vi "FTW-TestExecutive-Sequence-Serialize.vi"(0 "Sequence":T1[](array[typedef]) {"Results"."Start Time" format="%<%Y-%m-%d %H:%M:%S%03u>T"; "Results"."Elapsed Time" format="%<%H:%M:%S%3u>t"; "Elapsed Time" format="%<%H:%M:%S%3u>t"}, 11 "error in":errorcluster) -> (4 "JSON":string, 15 "error out":errorcluster)   [LabVIEW 2018]
doc: "Can be used to interpret the following messages\n\nSequenceLoaded\nSequenceComplete\nStepChange"
uses:
  FTW-TestExecutive-Step.ctl
  FTW-TestExecutive-Step-State.ctl
  FTW-TestExecutive-Results.ctl
  JSON/FTW-JSON-JoinMode.ctl
  c60d58ca-371a-4572-8f7b-04b3f362abcb.vi
  container/FTW-Container-FromVariant.vi
  container/FTW-Container-New-FromContainer.vi
  container/FTW-Container.lvclass
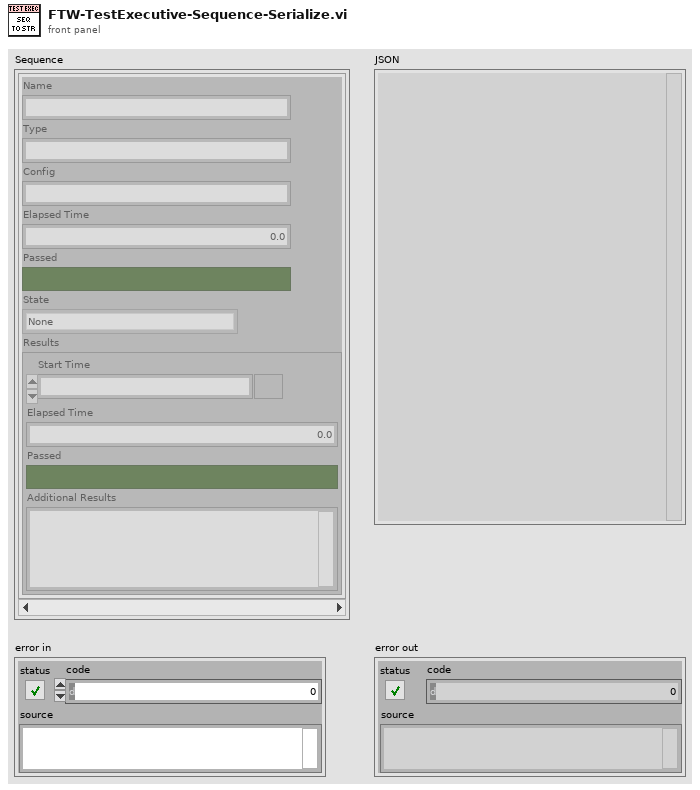
[diagram p1: front panel]
types:
  T1 = typedef "FTW-TestExecutive-Step.ctl" = cluster{"Name":string, "Type":string, "Config":string, "Elapsed Time":dbl, "Passed":bool, "State":T2, "Results":T3}
  T2 = typedef "FTW-TestExecutive-Step-State.ctl" = enum8{"None", "Failed", "Passed", "Timed out", "Aborted"}
  T3 = typedef "FTW-TestExecutive-Results.ctl" = cluster{"Start Time":timestamp, "Elapsed Time":dbl, "Passed":bool, "Additional Results":string}
  T4 = typedef "FTW-JSON-JoinMode.ctl" = enum32{"Upsert", "Update Only", "Insert Only"}
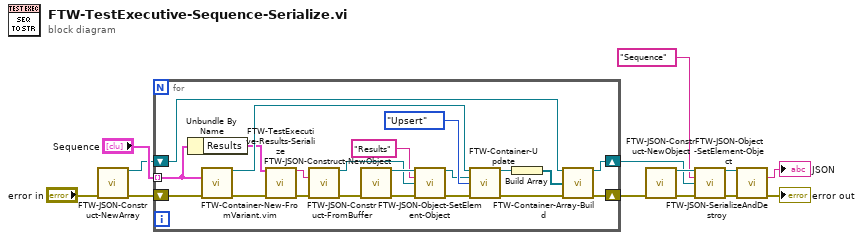
[diagram p0: block diagram]
diagram:
  n1 = call "FTW-JSON-Construct-NewArray.vi"("error in"="error in") -> ("JSON"=w9:refnum<class "FTW-Container.lvclass">, "error out"=w10:errorcluster)  [unwired: 13 in]
  n2 = for {
    tunnel: "Sequence" -> [w32] mode=indexing
    shift-right: [w23] -> w11
    shift-left: w10 -> [w24]
    shift-right: [w20] -> w5
    shift-left: w9 -> [w21]
    n3 = Unbundle By Name(w32) -> ("Results"=w30:T3)
    n4 = call "FTW-Container-New-FromVariant.vim"("Variant"=w32, "error in"=w24) -> ("FTW-Container"=w34:refnum<class "FTW-Container.lvclass">, "error out"=w28:errorcluster)  [unwired: 12 in]
    n5 = call "FTW-TestExecutive-Results-Serialize.vi"("Results"=w30, "error in (no error)"=w28) -> ("Serialized Results"=w31:string, "error out"=w29:errorcluster)  [unwired: 12 in]
    n6 = call "FTW-JSON-Construct-FromBuffer.vi"("JSON String (UTF-8)"=w31, "error in"=w29) -> ("JSON"=w15:refnum<class "FTW-Container.lvclass">, "error out"=w27:errorcluster)  [unwired: 12 in]
    n7 = call "FTW-JSON-Construct-NewObject.vi"("error in"=w27) -> ("JSON"=w17:refnum<class "FTW-Container.lvclass">, "error out"=w19:errorcluster)  [unwired: 13 in]
    n8 = call "FTW-JSON-Object-SetElement-Object.vi"("JSON Object"=w17, "Key"="Results", "JSON Sub-Object"=w15, "error in"=w19) -> ("JSON Root Object"=w16:refnum<class "FTW-Container.lvclass">, "error out"=w18:errorcluster)  [unwired: 10 in]
    n9 = call "FTW-Container-Update.vi"("FTW-Container In"=w34, "Other Container"=w16, "Join Mode"=FTW-JSON-JoinMode."Upsert", "error in"=w18) -> ("Updated Container"=w26:refnum<class "FTW-Container.lvclass">, "error out"=w22:errorcluster)  [unwired: 10 in]
    n10 = Build Array(w26) -> (w25:refnum<class "FTW-Container.lvclass">[])
    n11 = call "FTW-Container-Array-Build.vi"("FTW-Container In"=w21, "Array Elements"=w25, "error in"=w22) -> ("FTW-Container Out"=w20:refnum<class "FTW-Container.lvclass">, "error out"=w23:errorcluster)  [unwired: 11 in]
  }
  n12 = call "FTW-JSON-Construct-NewObject.vi"("error in"=w11) -> ("JSON"=w6:refnum<class "FTW-Container.lvclass">, "error out"=w8:errorcluster)  [unwired: 13 in]
  n13 = call "FTW-JSON-Object-SetElement-Object.vi"("JSON Object"=w6, "Key"="Sequence", "JSON Sub-Object"=w5, "error in"=w8) -> ("JSON Root Object"=w2:refnum<class "FTW-Container.lvclass">, "error out"=w7:errorcluster)  [unwired: 10 in]
  n14 = call "FTW-JSON-SerializeAndDestroy.vi"("JSON"=w2, "error in"=w7) -> ("JSON String (UTF-8)"=→"JSON":string, "error out"=→"error out":errorcluster)  [unwired: 12 in]
